vi "Write Conversion Time.vi"(8 "error in":errorcluster, 10 "conversion time":T1, 11 "analog input with conversion time mode in":refnum<class "Analog Input with Conversion Time Mode.lvclass">) -> (0 "error out":errorcluster, 3 "analog input with conversion time mode out":refnum<class "Analog Input with Conversion Time Mode.lvclass">)   [LabVIEW 2017, in "Scan Engine Scripting.lvlib" / "Analog Input with Conversion Time Mode.lvclass"]
uses:
  Analog Input with Conversion Time Mode.lvclass
  Conversion Time.ctl
  Analog Input with Conversion Time Mode.lvclass/Analog Input with Conversion Time Mode.ctl
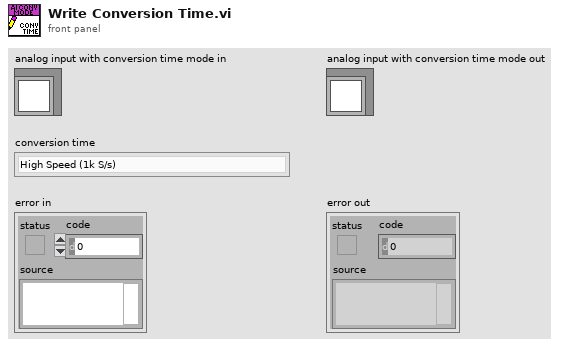
[diagram p1: front panel]
types:
  T1 = typedef "Scan Engine Scripting.lvlib/Analog Input with Conversion Time Mode.lvclass/Conversion Time.ctl" = enum16{"High Speed (1k S/s)", "Medium Speed (100 S/s)", "Medium Resolution (50/60Hz Rejection - 12 S/s)", "High Resolution (50/60Hz Rejection - 2 S/s)"}
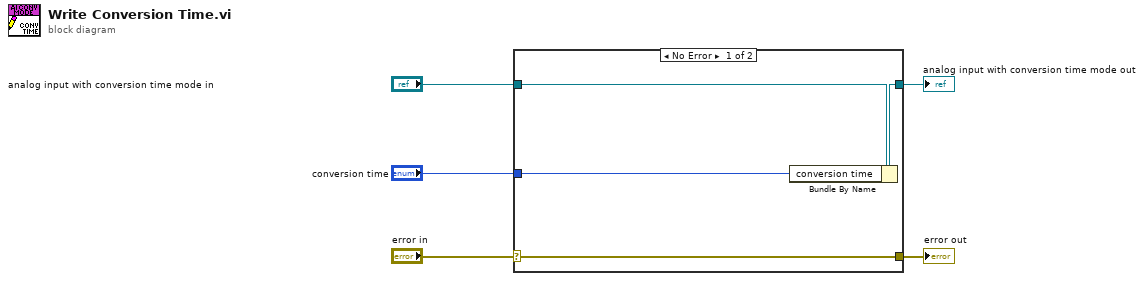
[diagram p0: block diagram]
diagram:
  n1 = case shown="No Error" "error in" {
    selector: "error in" -> [w9 w10]
    tunnel: [w9 w10] -> w4
    tunnel: [w7 w11] -> w2
    tunnel: "analog input with conversion time mode in" -> [w8 w11]
    tunnel: "conversion time" -> [w6 _]
    frame No Error {
      n2 = Bundle By Name(cluster=w8, "conversion time"=w6) -> (w7:refnum<class "Analog Input with Conversion Time Mode.lvclass">)
    }
    frame Error {
    }
  }
  "error out" <- w4
  "analog input with conversion time mode out" <- w2
